vi "Large Scan.vi"() -> ()   [LabVIEW 2020]
uses:
  Labview Library/Libraries/Basic Experiment/Basic Experiment.lvlib
  Labview Library/Libraries/PIScanner_new/Library/PIScanner.lvlib
  Labview Library/Libraries/Save Module/Libraries/Save Module/Save Module.lvlib
  Axis Enum.ctl
  Labview Library/Libraries/Basic Experiment/Scan Settings.ctl
  Labview Library/Libraries/LaoJi/UT_Utilities/Utilities.lvlib
  Labview Library/Libraries/Basic Experiment/1AutoTrace Settings.ctl
  Labview Library/Libraries/ExtraWork/Scan ExtraWork Settings.ctl
  Labview Library/Libraries/ExtraWork/ExtraWork Seq.ctl
  Labview Library/Libraries/ExtraWork/ExtraWork Seq.lvlib
  Labview Library/Libraries/ExtraWork/ExtraWork Additional Settings.ctl
  Labview Library/Libraries/Basic Experiment/CW settings.ctl
  Labview Library/Libraries/Basic Experiment/Rabi Settings.ctl
  Labview Library/Libraries/Basic Experiment/T1 Settings.ctl
  Labview Library/Libraries/Basic Experiment/Ramsey Settings.ctl
  Labview Library/Libraries/Basic Experiment/T2 Settings.ctl
panel:
  in  "Tab Control":T1(tab)
  out "Current Position":dbl[](array[numeric])=[120.006485, 9.997306824, 44.22160339]
  out "Z AutoTrace Graph":cluster{dbl[], dbl[]}[](graph)=[{[85.47172546, 85.71172546, 85.95172546, 86.19172546, 86.43172546, 86.67172546, 86.91172546, 87.15172546000001, 87.39172546, 87.63172546, 87.87172546000001, 88.11172546, 88.35172546, 88.59172546, 88.83172546, 89.07172546, 89.31172546, 89.55172546, 89.79172546000001, 90.03172546, 90.27172546, 90.51172546000001, 90.75172546, 90.99172546, 91.23172546, 91.47172546], [2392.2014233653763]}, {[85.47172546, 85.71172546, 85.95172546, 86.19172546, 86.43172546, 86.67172546, 86.91172546, 87.15172546000001, 87.39172546, 87.63172546, 87.87172546000001, 88.11172546, 88.35172546, 88.59172546, 88.83172546, 89.07172546, 89.31172546, 89.55172546, 89.79172546000001, 90.03172546, 90.27172546, 90.51172546000001, 90.75172546, 90.99172546, 91.23172546, 91.47172546], [233.553191646536]}]
  out "Intensity Graph":dbl[][](graph)
  in  "Stop Button":bool
  in  "Settings":T2={"Xstart"=120.0, "Xend"=180.0, "Xnum"=6, "Ystart"=10.0, "Yend"=50.0, "Ynum"=4}
  out "X step size":dbl=10.0
  out "Y step size":dbl=10.0
  in  "Extra Work Additional Settings":T3={"CW setting section"={"Num Pts"=50, "Start freq"=1310.0, "Stop freq"=1410.0, " dBm"=-12.0, "Loop times"=20000, "Ratio Thre(abs)"=0.04, "AutoTrace Before Exp"=FALSE, "RepoSave"=TRUE, "Peak Num Limit "=10}, "Cool Down Time(ms)"=3000, "Rabi settings"={"Num Pts"=30, "freq(MHz)"=1370.0, "dBm"=-2.0, "tau start"=0.0, "tau end"=2.5e-07, "Update Times"=100, "Loop per Update"=5000, "Channel Chooser"=enum."Channel X", "RepoSave"=TRUE, "AutoTrace Before Exp"=TRUE}, "T1 Settings"={"Pi(s)"=1.2e-07, "Loop Per Update"=2000, "Update Times"=250, "MW Fre"=1350.0, "MW Power"=-2.0, "Tau Start"=1e-07, "Tau End"=8e-05, "Num"=25, "AutoTrace Before Exp"=TRUE, "RepoSave"=TRUE}, "Ramsey Settings"={"1/2Pi(s)"=6e-08, "Loop Per Update"=20000, "Update Times"=250, "MW Fre"=1350.0, "MW Power"=-24.0, "Tau Start"=1e-08, "Tau End"=1e-06, "Num"=20, "AutoTrace Before Exp"=TRUE, "RepoSave"=TRUE, "3/2Pi(s)"=6e-08}, "T2 Settings"={"Loop Per Update"=40000, "Update Times"=250, "MW Fre"=1550.0, "MW Power"=-2.0, "Tau Start"=1e-07, "Tau End"=8e-06, "Num"=30, "1/2Pi(s)"=6e-08, "Pi(s)"=1.2e-07, "3/2Pi(s)"=6e-08, "AutoTrace Before Exp"=TRUE, "RepoSave"=TRUE}} {"T2 Settings"."3/2Pi(s)" format="%#_6p"; "T2 Settings"."Pi(s)" format="%#_6p"; "T2 Settings"."1/2Pi(s)" format="%#_6p"; "T2 Settings"."Tau End" format="%#_6p"; "T2 Settings"."Tau Start" format="%#_6p"; "Ramsey Settings"."3/2Pi(s)" format="%#_6p"; "Ramsey Settings"."Tau End" format="%#_6p"; "Ramsey Settings"."Tau Start" format="%#_6p"; "Ramsey Settings"."1/2Pi(s)" format="%#_6p"; "T1 Settings"."Tau End" format="%#_6p"; "T1 Settings"."Tau Start" format="%#_6p"; "T1 Settings"."Pi(s)" format="%#_6p"; "Rabi settings"."Loop per Update" format="%.0p"; "Rabi settings"."Update Times" format="%.0p"; "Rabi settings"."tau end" format="%#_6p"}
  in  "ExtraWork Settings":T9={"Extral Work Seq "=[enum."AutoTrace", enum."CW", enum."Cool Down", enum."Rabi", enum."Cool Down", enum."T2", enum."Cool Down", enum."T1", enum."AutoTrace", enum."Laser On"], "Threshold"=30000.0, "Max Points"=10} {"Threshold" format="%#_13g"}
  in  "Single axis Settings":T11={"Axis"=enum."z", "Sample Rate (Hz)"=20.0, "Diameter(um)"=6.0, "Num"=50, "Peak Threshold"=4000.0, "First Wait(ms)"=20, "Move wait(ms)"=20, "Final Wait(ms)"=50, "Read Final"=FALSE} {"Peak Threshold" format="%#_13g"}
  # "T2 Settings"
  # "Ramsey Settings"
  # "T1 Settings"
  # "Rabi Settings"
  # "CW Settings"
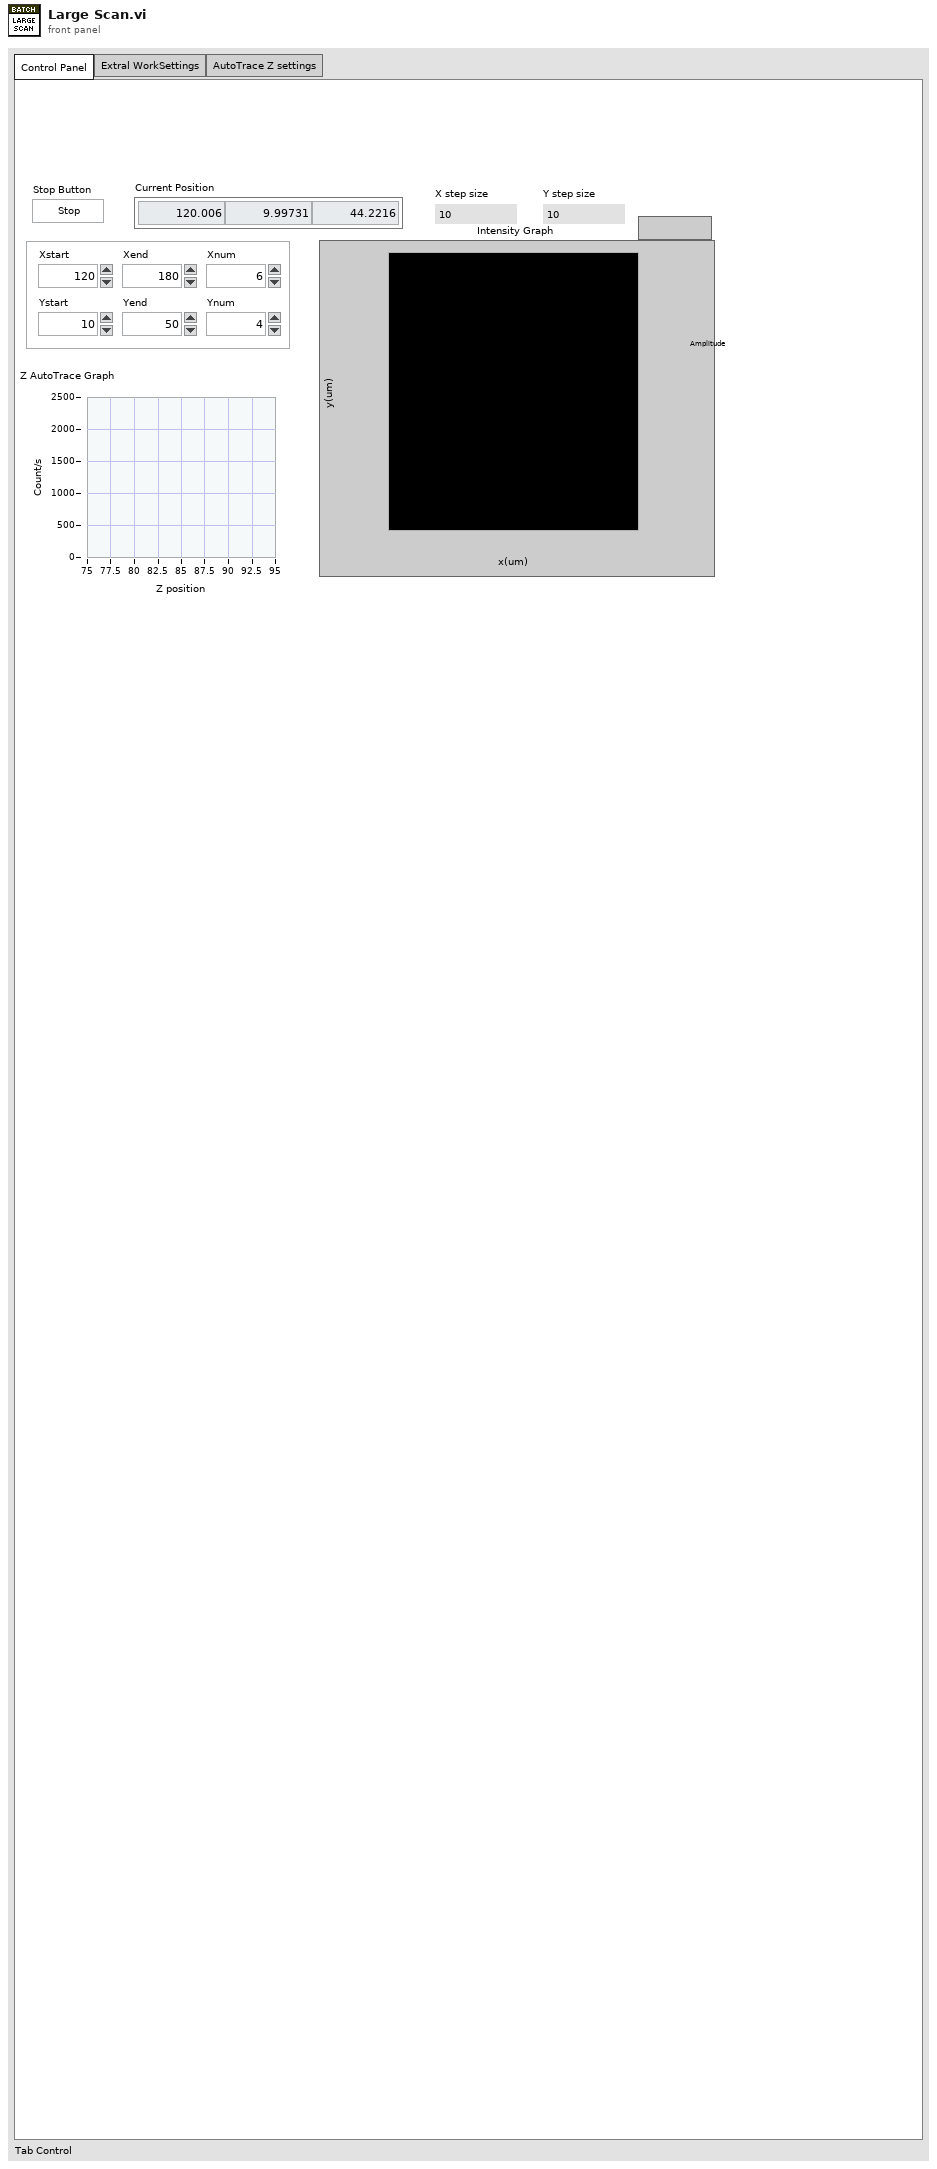
[diagram p1: front panel]
types:
  T1 = enum32{"Control Panel", "Extral WorkSettings", "AutoTrace Z settings"}
  T2 = cluster{"Xstart":dbl, "Xend":dbl, "Xnum":i32, "Ystart":dbl, "Yend":dbl, "Ynum":i32}
  T3 = typedef "ExtraWork Seq.lvlib/ExtraWork Additional Settings.ctl" = cluster{"CW setting section":T4, "Cool Down Time(ms)":u32, "Rabi settings":T5, "T1 Settings":T6, "Ramsey Settings":T7, "T2 Settings":T8}
  T4 = typedef "Basic Experiment.lvlib/CW settings.ctl" = cluster{"Num Pts":i32, "Start freq":dbl, "Stop freq":dbl, " dBm":dbl, "Loop times":i32, "Ratio Thre(abs)":dbl, "AutoTrace Before Exp":bool, "RepoSave":bool, "Peak Num Limit ":i32}
  T5 = typedef "Basic Experiment.lvlib/Rabi Settings.ctl" = cluster{"Num Pts":i32, "freq(MHz)":dbl, "dBm":dbl, "tau start":dbl, "tau end":dbl, "Update Times":u32, "Loop per Update":u32, "Channel Chooser":enum16{"Channel X", "Channel Y"}, "RepoSave":bool, "AutoTrace Before Exp":bool}
  T6 = typedef "Basic Experiment.lvlib/T1 Settings.ctl" = cluster{"Pi(s)":dbl, "Loop Per Update":u32, "Update Times":u32, "MW Fre":dbl, "MW Power":dbl, "Tau Start":dbl, "Tau End":dbl, "Num":u32, "AutoTrace Before Exp":bool, "RepoSave":bool}
  T7 = typedef "Basic Experiment.lvlib/Ramsey Settings.ctl" = cluster{"1/2Pi(s)":dbl, "Loop Per Update":u32, "Update Times":u32, "MW Fre":dbl, "MW Power":dbl, "Tau Start":dbl, "Tau End":dbl, "Num":u32, "AutoTrace Before Exp":bool, "RepoSave":bool, "3/2Pi(s)":dbl}
  T8 = typedef "Basic Experiment.lvlib/T2 Settings.ctl" = cluster{"Loop Per Update":u32, "Update Times":u32, "MW Fre":dbl, "MW Power":dbl, "Tau Start":dbl, "Tau End":dbl, "Num":u32, "1/2Pi(s)":dbl, "Pi(s)":dbl, "3/2Pi(s)":dbl, "AutoTrace Before Exp":bool, "RepoSave":bool}
  T9 = typedef "Basic Experiment.lvlib/Scan ExtraWork Settings.ctl" = cluster{"Extral Work Seq ":T10, "Threshold":dbl, "Max Points":i16}
  T10 = typedef "ExtraWork Seq.lvlib/ExtraWork Seq.ctl" = enum16{"T2", "T1", "Ramsey", "Rabi", "Laser On", "Cool Down", "CW", "Little Scan", "AutoTrace"}[]
  T11 = typedef "Basic Experiment.lvlib/1AutoTrace Settings.ctl" = cluster{"Axis":enum16{"x", "y", "z"}, "Sample Rate (Hz)":dbl, "Diameter(um)":dbl, "Num":i32, "Peak Threshold":dbl, "First Wait(ms)":u32, "Move wait(ms)":u32, "Final Wait(ms)":u32, "Read Final":bool}
  T12 = enum16{"Config Mode", "Slow Mode", "Test Mode", "Default Mode"}
  T13 = typedef "Basic Experiment.lvlib/Scan Settings.ctl" = cluster{"Vertical axis":T14, "Horizontal axis":T14, "vertical num":u32, "vertical end":dbl, "vertical start":dbl, "horizontal num":u32, "horizontal end":dbl, "horizontal start":dbl, "AutoTrace Z axis before Exp?":bool, "RepoSave":bool}
  T14 = typedef "Axis Enum.ctl" = enum16{"x", "y", "z"}
  T15 = typedef "Basic Experiment.lvlib/Scan Results.ctl" = cluster{"Intensity Graph":dbl[][], "ColorCenter in This Scan":T16[], "Tdms Path":path, "Image Path":path}
  T16 = typedef "Repository Control.lvlib/Single ColorCenter Element.ctl" = cluster{"Tdms Path":path, "Serial Num ":string, "Peak Count":dbl, "1/2pi":dbl, "pi":dbl, "3/2pi":dbl, "2pi":dbl, "Position":dbl[], "Fre1":T17, "Fre2":T17, "Fre3":T17, "MW Power for The Pulse":dbl, "T1":dbl, "Half T2":dbl, "1/2piy":dbl, "piy":dbl, "3/2piy":dbl, "2piy":dbl, "MW Power for The Pulse Y":dbl}
  T17 = typedef "Repository Control.lvlib/Frequency Control.ctl" = cluster{"Amplitude":dbl, "Position":dbl, "Width":dbl}
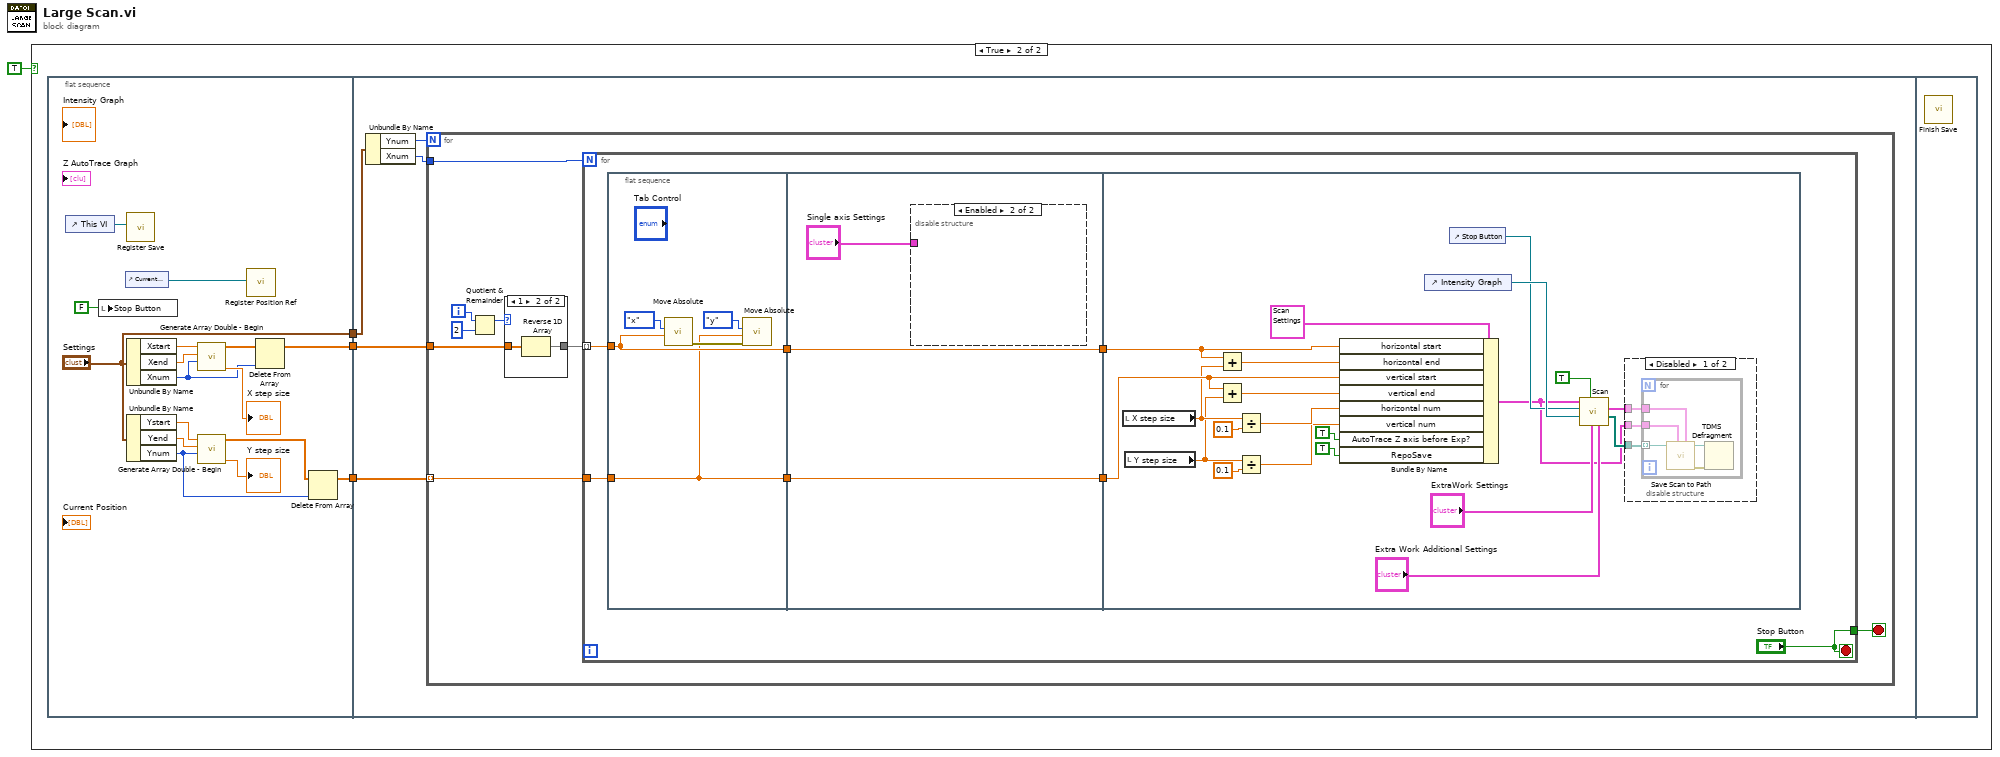
[diagram p0: block diagram]
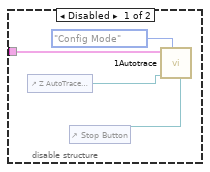
[diagram p4: hidden frame]
diagram:
  n1 = case shown="True" TRUE {
    frame False {
    }
    frame True {
      n2 = flat-sequence {
        tunnel: [w8] -> w4
        tunnel: [w5] -> w3
        tunnel: ["Settings"] -> w2
        tunnel: w4 -> [w25]
        tunnel: w3 -> [w24]
        tunnel: w2 -> [w23]
        frame #0 {
          n3 = control-ref of="This VI"() -> (w18:refnum<vi>)
          n4 = local write "Stop Button"(FALSE) -> ()
          n5 = control-ref of="Current Position"() -> (w19:refnum<vi>)
          n6 = call "Register Save.vi"("VI Refnum"=w18) -> ()  [unwired: 9 in, 2 out]
          n7 = Unbundle By Name("Settings") -> ("Xstart"=w17:dbl, "Xend"=w16:dbl, "Xnum"=w6:i32)
          n8 = Unbundle By Name("Settings") -> ("Ystart"=w15:dbl, "Yend"=w14:dbl, "Ynum"=w9:i32)
          n9 = call "Generate Array Double - Begin.vi"("num of step"=w6, "end"=w16, "begin"=w17) -> ("step size"=→"X step size":dbl, "output array"=w7:dbl[])  [unwired: 5 in, 2 out]
          n10 = call "Generate Array Double - Begin.vi"("num of step"=w9, "end"=w14, "begin"=w15) -> ("step size"=→"Y step size":dbl, "output array"=w10:dbl[])  [unwired: 5 in, 2 out]
          n11 = call "Register Position Ref.vi"("Current Position Ref"=w19) -> ()  [unwired: 10 in, 1 out]
          n12 = Delete From Array(array=w7, index=w6) -> (array with subset deleted=w5:dbl[])  [unwired: 1 in, 1 out]
          n13 = Delete From Array(array=w10, index=w9) -> (array with subset deleted=w8:dbl[])  [unwired: 1 in, 1 out]
        }
        frame #1 {
          n14 = Unbundle By Name(w23) -> ("Ynum"=w22:i32, "Xnum"=w21:i32)
          n15 = for {
            N: w22 -> [_]
            tunnel: w25 -> [w33] mode=indexing
            tunnel: w24 -> [w27]
            tunnel: w21 -> [w26]
            i -> [w31]
            stop <- w32 stop-if-true
            n16 = Quotient & Remainder(x=w31, y=2) -> (x-y*floor(x/y)=w29:i32)  [unwired: 1 out]
            n17 = case shown="1" w29 {
              tunnel: [w34 w35] -> w28
              tunnel: w27 -> [w34 w36]
              frame 0, Default {
              }
              frame 1 {
                n18 = Reverse 1D Array(array=w36) -> (reversed array=w35:dbl[])
              }
            }
            n19 = for {
              N: w26 -> [_]
              tunnel: w28 -> [w43] mode=indexing
              tunnel: w33 -> [w42]
              tunnel: ["Stop Button"] -> w32
              stop <- "Stop Button" stop-if-true
              n20 = flat-sequence {
                tunnel: w42 -> [w44]
                tunnel: w43 -> [w45]
                tunnel: [w45] -> w40
                tunnel: [w44] -> w38
                tunnel: w40 -> [w51]
                tunnel: [w51] -> w39
                tunnel: w38 -> [w50]
                tunnel: [w50] -> w37
                tunnel: w37 -> [w74]
                tunnel: w39 -> [w76]
                frame #0 {
                  n21 = call "Move Absolute.vi"("Goal Position"=w45, "Axis To Move"=enum16{"x", "y", "z"}."x") -> ("error out"=w46:errorcluster)  [unwired: 8 in, 1 out]
                  n22 = call "Move Absolute.vi"("error in"=w46, "Goal Position"=w44, "Axis To Move"=enum16{"x", "y", "z"}."y") -> ()  [unwired: 7 in, 2 out]
                }
                frame #1 {
                  n23 = disable-structure shown="Enabled" {
                    disable-tunnel: "Single axis Settings" -> [w52 _]
                    frame Disabled {
                      n24 = control-ref of="Z AutoTrace Graph"() -> (w55:refnum<vi>)
                      n25 = control-ref of="Stop Button"() -> (w54:refnum<vi>)
                      n26 = call "1Autotrace.vi"(4:w54, "Mode"=T12."Config Mode", "AutoTrace Graph"=w55, "Single axis Settings"=w52) -> ()  [unwired: 6 in, 2 out]
                    }
                    frame Enabled {
                    }
                  }
                }
                frame #2 {
                  n27 = local read "X step size"() -> (w65:dbl)
                  n28 = local read "Y step size"() -> (w64:dbl)
                  n29 = Add(x=w76, y=w65) -> (x+y=w75:dbl)
                  n30 = Add(x=w74, y=w64) -> (x+y=w73:dbl)
                  n31 = Divide(x=w65, y=0.1) -> (x/y=w67:dbl)
                  n32 = Divide(x=w64, y=0.1) -> (x/y=w66:dbl)
                  n33 = Bundle By Name(cluster=T13 {"Vertical axis"=enum."y", "Horizontal axis"=enum."x", "vertical num"=100, "vertical end"=50.0, "vertical start"=40.0, "horizontal num"=100, "horizontal end"=25.0, "horizontal start"=15.0, "AutoTrace Z axis before Exp?"=FALSE, "RepoSave"=FALSE} ("Scan parameter"), "horizontal start"=w76, "horizontal end"=w75, "vertical start"=w74, "vertical end"=w73, "horizontal num"=w67, "vertical num"=w66, "AutoTrace Z axis before Exp?"=TRUE, "RepoSave"=TRUE) -> (w58:T13)
                  n34 = control-ref of="Intensity Graph"() -> (w72:refnum<vi>)
                  n35 = control-ref of="Stop Button"() -> (w71:refnum<vi>)
                  n36 = call "Scan.vi"("Extra Work Additional Settings"="Extra Work Additional Settings", "ExtraWork Settings"="ExtraWork Settings", "Extral Work"=TRUE, "Intensity Graph Ref"=w72, 10:w71, "Scan Settings"=w58) -> ("Tdms Array"=w60:path[], "Scan Results"=w57:T15)  [unwired: 3 in, 1 out]
                  n37 = disable-structure shown="Disabled" {
                    disable-tunnel: w60 -> [w79 _]
                    disable-tunnel: w58 -> [w78 _]
                    disable-tunnel: w57 -> [w77 _]
                    frame Disabled {
                      n38 = for {
                        tunnel: w78 -> [w81]
                        tunnel: w79 -> [w84] mode=indexing
                        tunnel: w77 -> [w80]
                        n39 = call "Save Scan to Path.vi"("Scan Results"=w80, "Scan Settings"=w81, "file path"=w84) -> ("error out"=w83:errorcluster, "file path out"=w82:path)  [unwired: 5 in, 2 out]
                        n40 = TDMS Defragment(4:w83, 7:w82) -> ()  [unwired: 1 out]
                      }
                    }
                    frame Enabled {
                    }
                  }
                }
              }
            }
          }
        }
        frame #2 {
          n41 = call "Finish Save.vi"() -> ()  [unwired: 11 in, 1 out]
        }
      }
    }
  }
